vi "Untitled 1.vi"() -> ()   [LabVIEW 2014, in "Lutron QS Control Protocol.lvlib" / "Lutron QS Object.lvclass"]
uses:
  Lutron QS Object.lvclass
panel:
  out "Array 2":i32[](array[numeric])
  out "Array":string[](array[string])
  out "return count":u32
  out "read buffer":string
  out "length":i32
  out "Numeric Control":i32
  out "error out":errorcluster
  in  "VISA resource name":refnum<visa-resource-name>
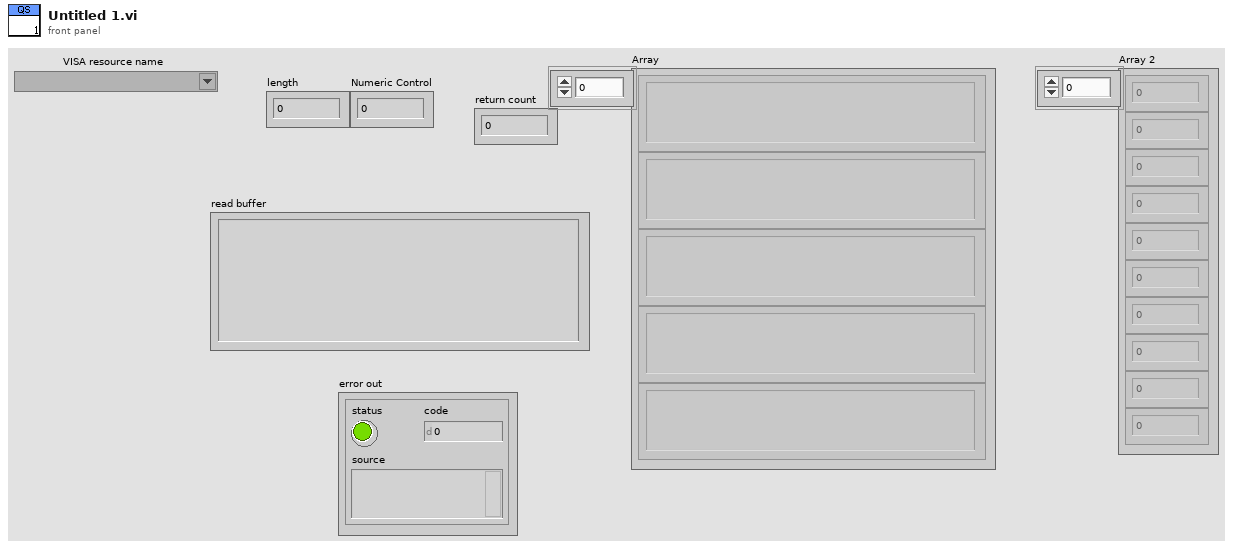
[diagram p1: front panel]
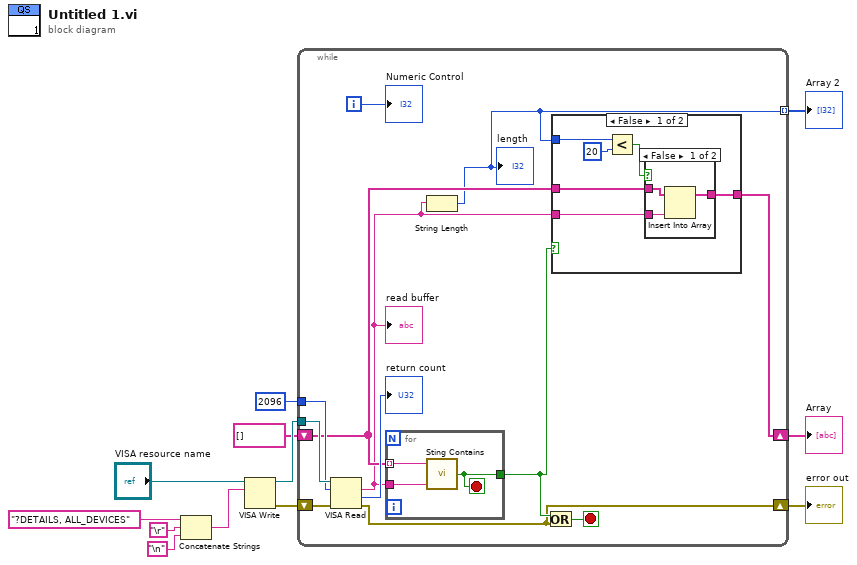
[diagram p0: block diagram]
diagram:
  n1 = Concatenate Strings("?DETAILS, ALL_DEVICES" ("string"), "\r", "\n") -> (w9:string)
  n2 = VISA Write(VISA resource name="VISA resource name", write buffer=w9) -> (VISA resource name out=w12:refnum<visa-resource-name>, error out=w11:errorcluster)  [unwired: 1 in, 1 out]
  n3 = while {
    tunnel: w12 -> [w24]
    shift-right: [w15] -> w10
    shift-left: w11 -> [w23]
    tunnel: u32 2096 ("byte count") -> [w20]
    shift-right: [w17] -> w2
    shift-left: string[] [] -> [w19]
    tunnel: [w13] -> w1 mode=indexing
    i -> [w21]
    stop <- w14 stop-if-true
    n4 = VISA Read(VISA resource name=w24, byte count=w20, error in (no error)=w23) -> (read buffer=w18:string, return count=→"return count":u32, error out=w15:errorcluster)  [unwired: 1 out]
    "read buffer" <- w18
    n5 = for {
      tunnel: [w38] -> w16
      tunnel: w19 -> [w37] mode=indexing
      tunnel: w18 -> [w36]
      stop <- w38 stop-if-true
      n6 = call "Sting Contains.vi"("Regular expression"=w36, "Input String"=w37) -> ("Boolean"=w38:bool)  [unwired: 3 in]
    }
    n7 = String Length(string=w18) -> (length=w13:i32)
    "length" <- w13
    n8 = Or(x=w16, y=w15) -> (x .or. y?=w14:bool)
    n9 = case shown="False" w16 {
      tunnel: w19 -> [w30 w35]
      tunnel: w18 -> [w29 _]
      tunnel: [w28 w35] -> w17
      tunnel: w13 -> [w27 _]
      frame False {
        n10 = Less?(x=w27, y=20) -> (x < y?=w25:bool)
        n11 = case shown="False" w25 {
          tunnel: w30 -> [w33 w34]
          tunnel: w29 -> [w32 _]
          tunnel: [w31 w34] -> w28
          frame False {
            n12 = Insert Into Array(array=w33, new element=w32) -> (w31:string[])  [unwired: 1 in]
          }
          frame True {
          }
        }
      }
      frame True {
      }
    }
    "Numeric Control" <- w21
  }
  "error out" <- w10
  "Array" <- w2
  "Array 2" <- w1
